vi "Create File.vi"(8 "error in":errorcluster, 10 "DirectoryPath":string, 11 "Part Number":string) -> (0 "error out":errorcluster, 3 "File Path Control":path)   [LabVIEW 2017]
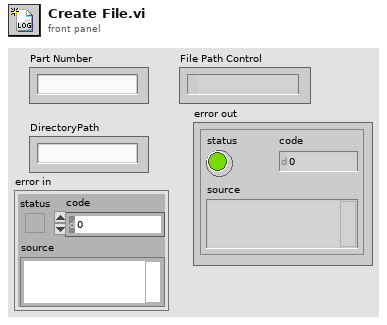
[diagram p1: front panel]
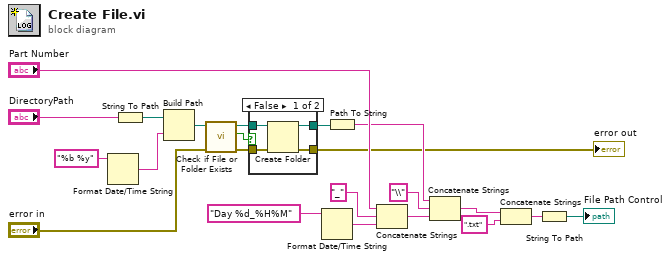
[diagram p0: block diagram]
diagram:
  n1 = Format Date/Time String(time format string (%c)="%b %y") -> (date/time string=w15:string)  [unwired: 2 in]
  n2 = String To Path(string="DirectoryPath") -> (path=w14:path)
  n3 = Build Path(base path=w14, name or relative path=w15) -> (appended path=w8:path)
  n4 = call <vilib>:"Check if File or Folder Exists.vi"("error in (no error)"="error in", "path"=w8) -> ("error out"=w2:errorcluster, "file or folder exists?"=w10:bool, "dup path"=w9:path)  [unwired: 7 in]
  n5 = case shown="False" w10 {
    tunnel: w9 -> [w26 w28]
    tunnel: [w25 w28] -> w12
    tunnel: w2 -> [w24 w27]
    tunnel: [w23 w27] -> w1
    frame False {
      n6 = Create Folder(path (use dialog)=w26, error in=w24) -> (created path=w25:path, error out=w23:errorcluster)  [unwired: 1 in, 1 out]
    }
    frame True {
    }
  }
  "error out" <- w1
  n7 = Format Date/Time String(time format string (%c)="Day %d_%H%M") -> (date/time string=w5:string)  [unwired: 2 in]
  n8 = Path To String(path=w12) -> (string=w13:string)
  n9 = Concatenate Strings("Part Number", "_" ("string"), w5) -> (w4:string)
  n10 = Concatenate Strings(w13, "\\" ("string"), w4) -> (w6:string)
  n11 = Concatenate Strings(w6, ".txt" ("string")) -> (w7:string)
  n12 = String To Path(string=w7) -> (path=→"File Path Control":path)
